vi "serial_baudrate.vi"(11 "baud rate":i32(ring)=10 items=["300", "1200", "2400", "4800", "9600", "14400", "19200", "28800", "38400", "57600", "115200", "230400"]) -> (8 "tick/2 every bit":u32, 10 "tick every bit":u32, 15 "tick after stop bit":u32)   [LabVIEW 2015]
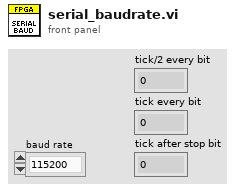
[diagram p1: front panel]
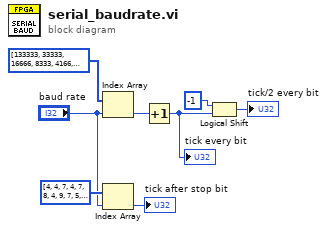
[diagram p0: block diagram]
diagram:
  n1 = Index Array(array=u32[] [133333, 33333, 16666, 8333, 4166, 2777, 2083, 1388, 1041, 694, 347, 173] ("32bit integer 2"), index="baud rate") -> (element=w6:u32)
  n2 = Index Array(array=u32[] [4, 4, 7, 4, 7, 8, 4, 9, 7, 5, 3, 7] ("32bit integer 3"), index="baud rate") -> (element=→"tick after stop bit":u32)
  n3 = Increment(x=w6) -> (x+1=w5:u32)
  "tick every bit" <- w5
  n4 = Logical Shift(y=i16 -1, x=w5) -> (x << y=→"tick/2 every bit":u32)
